vi "Status (Read).vi"(6 "ISOBUS address":T3=-1 caption="ISOBUS address (-1)", 8 "error in":errorcluster, 10 "Output to Read":u8, 11 "Mercury Reference In":T4) -> (0 "error out":errorcluster, 2 "State":T1, 3 "Mercury Reference Out":T4, 4 "Valid?":T2)   [LabVIEW 2016]
doc: "Read the output state of an output."
uses:
  Controls/Mercury Reference.ctl
  Controls/Comms Transport Layer.ctl
  Private/Controls/Query Dynamic Reference.ctl
  Controls/ISOBus Address.ctl
  Controls/Is Valid LED.ctl
  Controls/Unit String.ctl
  Private/Controls/Command Verbs.ctl
  Mercury iXX.lvlib
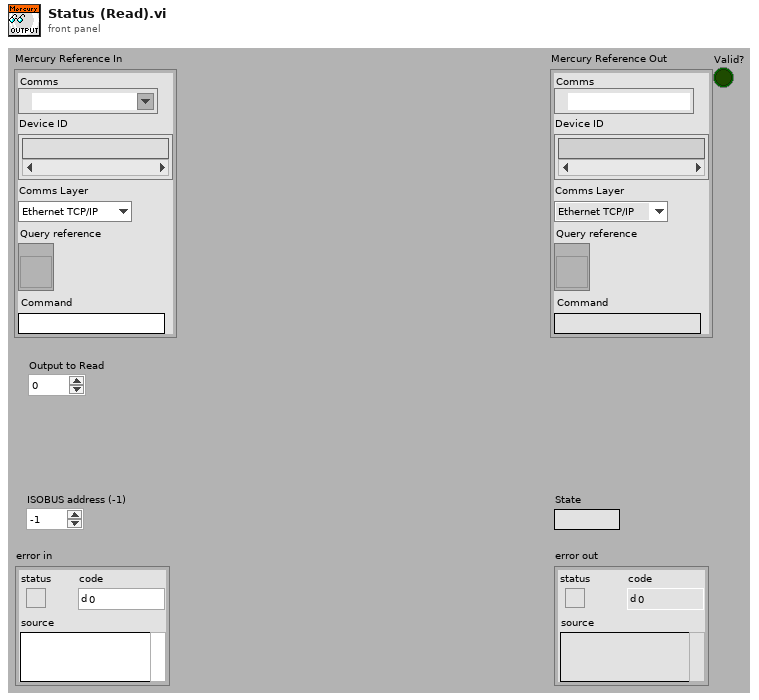
[diagram p1: front panel]
types:
  T1 = typedef "Mercury iXX.lvlib/Unit String.ctl" = string
  T2 = typedef "Mercury iXX.lvlib/Is Valid LED.ctl" = bool
  T3 = typedef "Mercury iXX.lvlib/ISOBus Address.ctl" = i32
  T4 = typedef "Mercury iXX.lvlib/Mercury Reference.ctl" = cluster{"Comms":refnum<visa-resource-name>, "Device ID":string[], "Comms Layer":T5, "Command":string, "Query reference":T6}
  T5 = typedef "Mercury iXX.lvlib/Comms Transport Layer.ctl" = enum16{"Ethernet TCP/IP", "USB", "ISOBus - RS-232", "GPIB"}
  T6 = typedef "Mercury iXX.lvlib/Query Dynamic Reference.ctl" = refnum<vi>
  T7 = typedef "Mercury iXX.lvlib/Command Verbs.ctl" = string
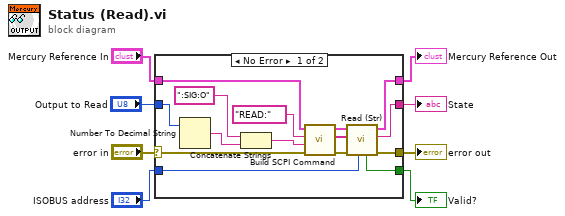
[diagram p0: block diagram]
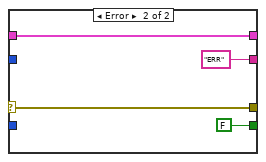
[diagram p2: hidden frame]
diagram:
  n1 = case shown="No Error" "error in" {
    selector: "error in" -> [w17 w26]
    tunnel: "Mercury Reference In" -> [w18 w27]
    tunnel: [w23 w26] -> w3
    tunnel: [w22 w27] -> w5
    tunnel: "ISOBUS address" -> [w21 _]
    tunnel: [w20 T2 FALSE ("Valid?")] -> w4
    tunnel: [w19 T1 "ERR" ("Unit")] -> w2
    tunnel: "Output to Read" -> [w11 _]
    frame No Error {
      n2 = Number To Decimal String(number=w11) -> (decimal integer string=w9:string)  [unwired: 1 out]
      n3 = Concatenate Strings(":SIG:O" ("Command"), w9) -> (w10:string)
      n4 = call "Build SCPI Command.vi"("error in"=w17, "Noun(s)"=w10, "Verb"=T7 "READ:", "Mercury Reference In"=w18) -> ("error out"=w13:errorcluster, "SCPI Message(s)"=w12:string[], "Mercury Reference Out"=w16:T4)  [unwired: 5 out]
      n5 = call "Read (Str).vi"("ISOBUS address"=w21, "error in"=w13, "SCPI Message(s)"=w12, "Mercury Reference In"=w16) -> ("error out"=w23:errorcluster, "Response"=w19:string, "Mercury Reference Out"=w22:T4, "Valid?"=w20:T2)  [unwired: 4 out]
    }
    frame Error {
    }
  }
  "Mercury Reference Out" <- w5
  "Valid?" <- w4
  "error out" <- w3
  "State" <- w2
